vi "Lambda_tau,T,W 1(s').vi"(6 "k":i32, 8 "w":dbl, 9 "T":dbl, 10 "t":dbl, 11 "s'":dbl) -> (3 "L_t,T,W(s')":dbl)   [LabVIEW 2021, in "Phasor.lvlib"]
uses:
  Phasor/Phasor.lvlib
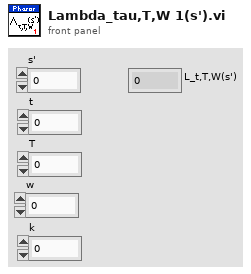
[diagram p1: front panel]
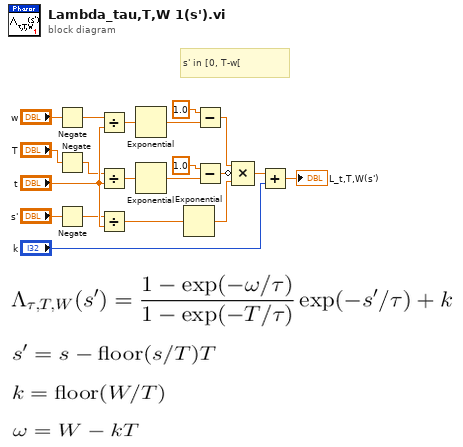
[diagram p0: block diagram]
diagram:
  # "s' in [0, T-w["
  n1 = Negate(x="w") -> (-x=w19:dbl)
  n2 = Negate(x="T") -> (-x=w13:dbl)
  n3 = Negate(x="s'") -> (-x=w8:dbl)
  n4 = Divide(x=w19, y="t") -> (x/y=w17:dbl)
  n5 = Divide(x=w13, y="t") -> (x/y=w12:dbl)
  n6 = Divide(x=w8, y="t") -> (x/y=w7:dbl)
  n7 = Exponential(1:w17) -> (0:w15:dbl)
  n8 = Exponential(1:w12) -> (0:w10:dbl)
  n9 = Exponential(1:w7) -> (0:w6:dbl)
  n10 = Subtract(x=1.0, y=w15) -> (x-y=w2:dbl)
  n11 = Subtract(x=1.0, y=w10) -> (x-y=w1:dbl)
  n12 = Compound Arithmetic op=MULTIPLY(w2, invert w1, w6) -> (w3:dbl)
  n13 = Add(x=w3, y="k") -> (x+y=→"L_t,T,W(s')":dbl)
